vi "Stop Test.vi"(6 "timeout (ms)":i32=-1, 8 "error in (no error)":errorcluster, 11 "FlexLogger_gRPCAPI in":refnum<class "FlexLogger_gRPC.lvclass">) -> (0 "error out":errorcluster, 3 "FlexLogger_gRPCAPI out":refnum<class "FlexLogger_gRPC.lvclass">)   [LabVIEW 2020, in "FlexLogger_gRPC.lvlib" / "FlexLogger_gRPC.lvclass"]
doc: "Stops the current test session in flexlogger"
uses:
  FlexLogger_gRPC.lvclass
  FlexLogger_gRPC.lvclass/FlexLogger_gRPC.ctl
  FlexLogger_client/FlexLogger_client.lvlib
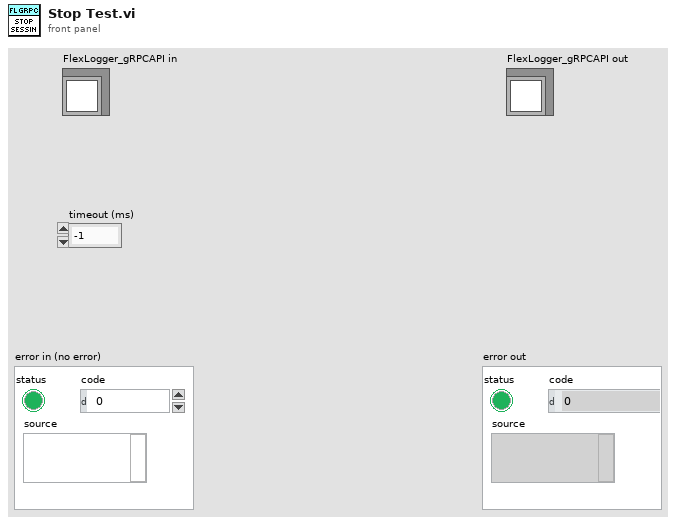
[diagram p1: front panel]
types:
  T1 = typedef "grpc-lvsupport-release.lvlib/grpcId.ctl" = u64
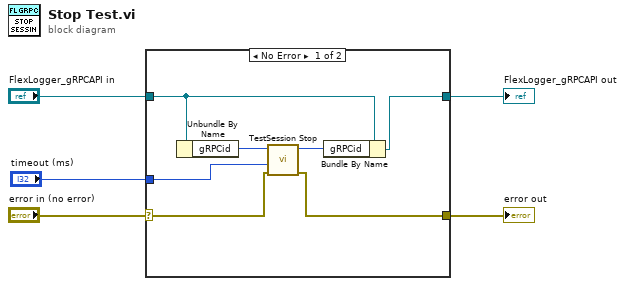
[diagram p0: block diagram]
diagram:
  n1 = case shown="No Error" "error in (no error)" {
    selector: "error in (no error)" -> [w8 w13]
    tunnel: "FlexLogger_gRPCAPI in" -> [w11 w14]
    tunnel: [w10 w14] -> w4
    tunnel: [w7 w13] -> w2
    tunnel: "timeout (ms)" -> [w6 _]
    frame No Error {
      n2 = Unbundle By Name(w11) -> ("gRPCid"=w12:T1)
      n3 = call "TestSession Stop.vi"("error in"=w8, "timeout (ms)"=w6, "gRPC ID"=w12) -> ("error out"=w7:errorcluster, "gRPC ID out"=w9:T1)  [unwired: 6 in, 1 out]
      n4 = Bundle By Name(cluster=w11, "gRPCid"=w9) -> (w10:refnum<class "FlexLogger_gRPC.lvclass">)
    }
    frame Error {
    }
  }
  "error out" <- w2
  "FlexLogger_gRPCAPI out" <- w4
